vi "main.vi"   [LabVIEW 2011]
uses:
  030 - EVENTS/EnumFgvEventCommand.ctl
  040 - SCREENS/enumScreen.ctl
  <vilib>/Utility/error.llb/DialogType.ctl
  090 - ERRORS/Ctrls/enumLogAndView.ctl
panel:
  # "MAIN"
types:
  T1 = typedef "EnumFgvEventCommand.ctl" = enum16{"Setup", "Cleanup", "Get"}
  T2 = enum32{"Invalid", "Standard", "Closed", "Hidden", "Minimized", "Maximized"}
  T3 = typedef "enumLogAndView.ctl" = enum16{"Log only", "Log and view"}
  T4 = typedef "enumScreen.ctl" = enum16{"Test screen", "Ecran principal", "LOG", "Setup", "Popup : About", "Popup : View last message", "Popup : WebBrowser help", "Traduction", "Popup : DEBUG Process"}
  T5 = typedef "DialogType.ctl" = u16
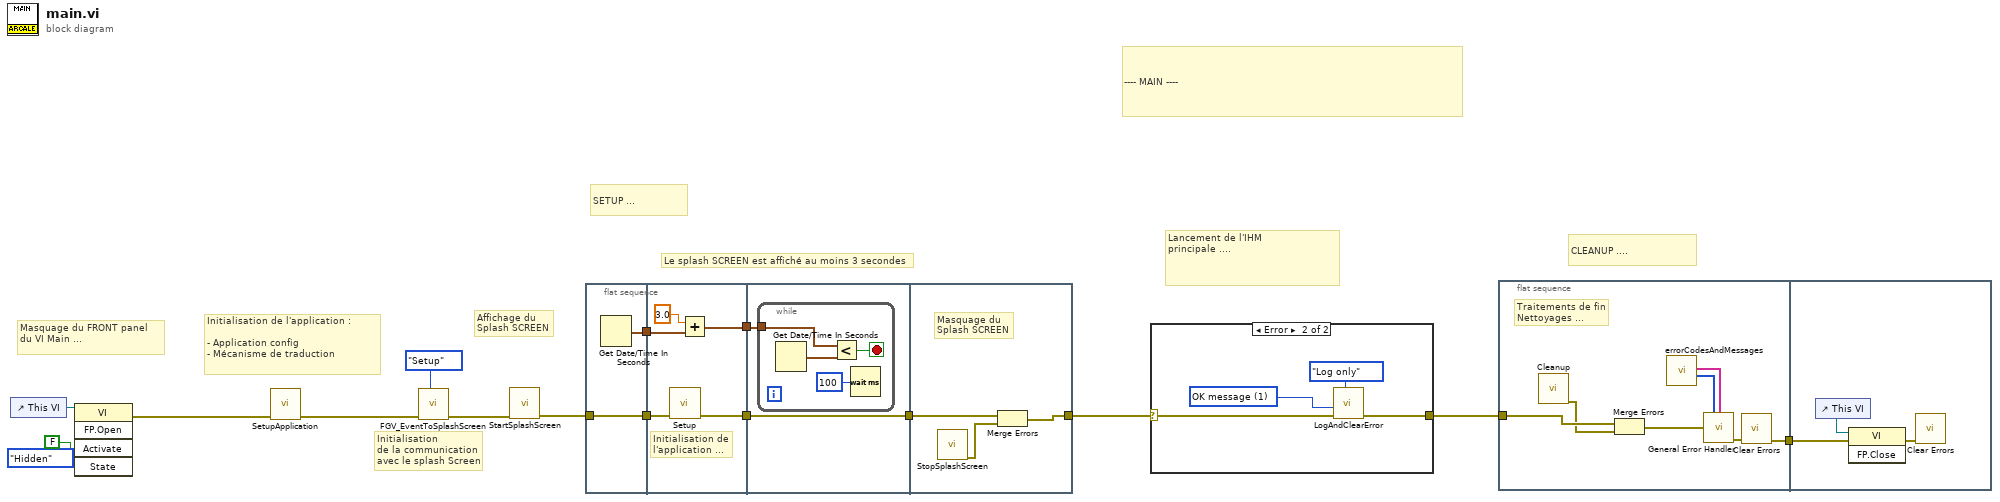
[diagram p0: block diagram]
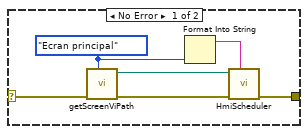
[diagram p2: hidden frame]
diagram:
  # "Initialisation de l'application :\n\n- Application config\n- Mécanisme de traduction"
  # "CLEANUP ...."
  # "SETUP ..."
  # "Le splash SCREEN est affiché au moins 3 secondes"
  # "Lancement de l'IHM\nprincipale ...."
  # "Initialisation\nde la communication\navec le splash Screen"
  # "Masquage du FRONT panel\ndu VI Main ..."
  # "Affichage du\nSplash SCREEN"
  # "---- MAIN ----"
  n1 = control-ref of="This VI"() -> (w16:refnum<vi>)
  n2 = invoke class="VI" method="FP.Open"(reference=w16, "Activate"=FALSE ("Activate?"), "State"=T2."Hidden") -> (error out=w5:errorcluster)  [unwired: 2 in, 4 out]
  n3 = call "SetupApplication.vi"("error in (no error)"=w5) -> ("error out"=w4:errorcluster)  [unwired: 10 in]
  n4 = call "FGV_EventToSplashScreen.vi"("Command"=EnumFgvEventCommand."Setup", "error in (no error)"=w4) -> ("error out"=w3:errorcluster)  [unwired: 8 in, 1 out]
  n5 = call "StartSplashScreen.vi"("error in (no error)"=w3) -> ("error out"=w2:errorcluster)  [unwired: 10 in]
  n6 = flat-sequence {
    tunnel: w2 -> [w18]
    tunnel: [w18] -> w12
    tunnel: [w17] -> w11
    tunnel: w12 -> [w23]
    tunnel: w11 -> [w22]
    tunnel: [w20] -> w10
    tunnel: [w19] -> w1
    tunnel: w10 -> [w25]
    tunnel: [w24] -> w8
    tunnel: w1 -> [w24]
    tunnel: [w31] -> w6
    tunnel: w8 -> [w32]
    frame #0 {
      n7 = Get Date/Time In Seconds() -> (seconds since 1Jan1904=w17:timestamp)
    }
    frame #1 {
      # "Initialisation de\nl'application ..."
      n8 = call "Setup.vi"("error in (no error)"=w23) -> ("error out"=w19:errorcluster)  [unwired: 10 in]
      n9 = Add(x=3.0, y=w22) -> (x+y=w20:timestamp)
    }
    frame #2 {
      n10 = while {
        tunnel: w25 -> [w27]
        stop <- w29 stop-if-true
        n11 = Get Date/Time In Seconds() -> (seconds since 1Jan1904=w28:timestamp)
        n12 = Less?(x=w27, y=w28) -> (x < y?=w29:bool)
        n13 = Wait (ms)(milliseconds to wait=u32 100) -> ()  [unwired: 1 out]
      }
    }
    frame #3 {
      # "Masquage du\nSplash SCREEN"
      n14 = call "StopSplashScreen.vi"() -> ("error out"=w30:errorcluster)  [unwired: 11 in]
      n15 = Merge Errors(w32, w30) -> (w31:errorcluster)
    }
  }
  n16 = case shown="Error" w6 {
    selector: w6 -> [w33 w41]
    tunnel: [w34 w42] -> w9
    frame No Error {
      w36 = enumScreen."Ecran principal" ("Enum Screen")
      n17 = call "getScreenViPath.vi"("Enum Screen"=w36, "error in (no error)"=w33) -> ("error out"=w38:errorcluster, "Path"=w37:path)  [unwired: 8 in]
      n18 = Format Into String(w36) -> (resulting string=w35:string)  [unwired: 3 in, 1 out]
      n19 = call "HmiScheduler.vi"("Param Screen Title"=w35, "error in (no error)"=w38, "Param Initial VI Path"=w37) -> ("error out"=w34:errorcluster)  [unwired: 8 in]
    }
    frame Error {
      w39 = T5 1 items=["no dialog", "OK message", "continue or stop message", "OK message + warnings", "continue/stop + warnings"] ("type of dialog")
      n20 = call "LogAndClearError.vi"("Log and view ?"=enumLogAndView."Log only", "error in (no error)"=w41, "type of dialog"=w39) -> ("error out"=w42:errorcluster)  [unwired: 8 in]
    }
  }
  n21 = flat-sequence {
    tunnel: [w43] -> w7
    tunnel: w9 -> [w49]
    tunnel: w7 -> [w51]
    frame #0 {
      # "Traitements de fin\nNettoyages ..."
      n22 = call "Cleanup.vi"() -> ("error out"=w48:errorcluster)  [unwired: 11 in]
      n23 = Merge Errors(w49, w48) -> (w47:errorcluster)
      n24 = call "errorCodesAndMessages.vi"() -> ("errorCodes"=w45:i32[], "errorMessages"=w46:string[])  [unwired: 10 in]
      n25 = call <vilib>:"General Error Handler.vi"("[user-defined codes]"=w45, "[user-defined descriptions]"=w46, "error in (no error)"=w47) -> ("error out"=w44:errorcluster)  [unwired: 8 in, 4 out]
      n26 = call <vilib>:"Clear Errors.vi"("error in (no error)"=w44) -> ("error out"=w43:errorcluster)  [unwired: 6 in]
    }
    frame #1 {
      n27 = control-ref of="This VI"() -> (w52:refnum<vi>)
      n28 = invoke class="VI" method="FP.Close"(reference=w52, error in=w51) -> (error out=w50:errorcluster)  [unwired: 1 in, 2 out]
      n29 = call <vilib>:"Clear Errors.vi"("error in (no error)"=w50) -> ()  [unwired: 6 in, 1 out]
    }
  }
